vi "OE1022D_Configure_Setting.vi"(0 "VISA resource name":refnum<visa-resource-name>, 1 "Read SET":bool, 2 "Save SET":bool, 3 "error in (no error)":errorcluster, 4 "Menu":u16(ring) items=["默认设置", "设置1", "设置2", "设置3", "设置4"]) -> (5 "VISA resource name out":refnum<visa-resource-name>, 6 "error out":errorcluster)   [LabVIEW 2021]
doc: "Configures the reference source and the internal oscillator."
uses:
  <vilib>/Instr/_visa.llb/VISA Flush IO Buffer Mask.ctl
panel:
  in  "连接的字符串":string
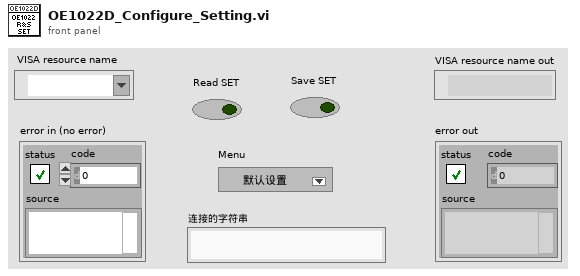
[diagram p1: front panel]
types:
  T1 = typedef "VISA Flush IO Buffer Mask.ctl" = u16
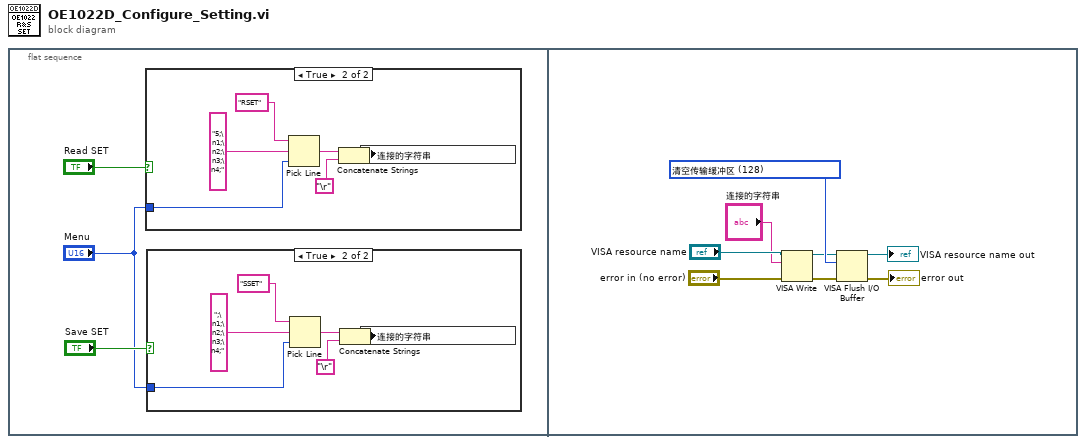
[diagram p0: block diagram]
diagram:
  n1 = flat-sequence {
    frame #0 {
      n2 = case shown="True" "Read SET" {
        tunnel: "Menu" -> [_ w4]
        frame False {
        }
        frame True {
          n3 = Pick Line(string ("")="RSET" ("字符串(\"\")"), multi-line string="5;\n1;\n2;\n3;\n4;" ("多行字符串"), line index=w4) -> (output string=w8:string)
          n4 = Concatenate Strings(w8, "\r") -> (w5:string)
          n5 = local write "连接的字符串"(w5) -> ()
        }
      }
      n6 = case shown="True" "Save SET" {
        tunnel: "Menu" -> [_ w10]
        frame False {
        }
        frame True {
          n7 = Pick Line(string ("")="SSET" ("字符串(\"\")"), multi-line string=";\n1;\n2;\n3;\n4;" ("多行字符串"), line index=w10) -> (output string=w14:string)
          n8 = Concatenate Strings(w14, "\r") -> (w11:string)
          n9 = local write "连接的字符串"(w11) -> ()
        }
      }
    }
    frame #1 {
      w20 = T1 128 items=["清空接收缓冲区"=16, "向设备写入传输缓冲区"=32, "清空接收缓冲区（无I/O）"=64, "清空传输缓冲区"=128] ("Mask")
      n10 = VISA Write(VISA resource name="VISA resource name", write buffer="连接的字符串", error in (no error)="error in (no error)") -> (VISA resource name out=w19:refnum<visa-resource-name>, error out=w18:errorcluster)  [unwired: 1 out]
      n11 = VISA Flush I/O Buffer(VISA resource name=w19, mask (16)=w20, error in (no error)=w18) -> (VISA resource name out=→"VISA resource name out":refnum<visa-resource-name>, error out=→"error out":errorcluster)
    }
  }
